vi "VelocityMeasure.vi"(5 "On/Off":bool, 6 "error in (no error)":errorcluster, 7 "Gray Image":T2, 8 "曝光时间/us":dbl, 9 "dpp/um":dbl) -> (0 "error out":errorcluster, 1 "粒子速度分布图":cluster{dbl[], i32[]}, 2 "实时速度":T1, 3 "平均速度":dbl format="%0.2f")   [LabVIEW 2012]
uses:
  <vilib>/vision/Image Controls.llb/IMAQ Image.ctl
  <vilib>/vision/NI_Vision_Development_Module.lvlib
  <vilib>/gmath/NI_Gmath.lvlib
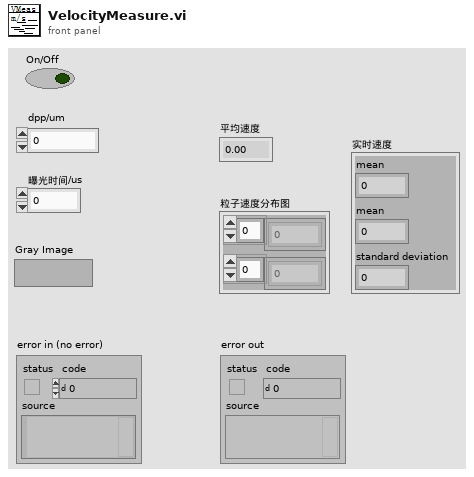
[diagram p1: front panel]
types:
  T1 = cluster{"mean":dbl, "mean":dbl, "standard deviation":dbl}
  T2 = typedef "IMAQ Image.ctl" = refnum<image>
  T3 = enum16{"arithmetic", "geometric", "harmonic", "trimmed", "median"}
  T4 = typedef "Particle Parameters" = i32
  T5 = cluster{"mean value":dbl, "mean value":dbl, "spread value":dbl}
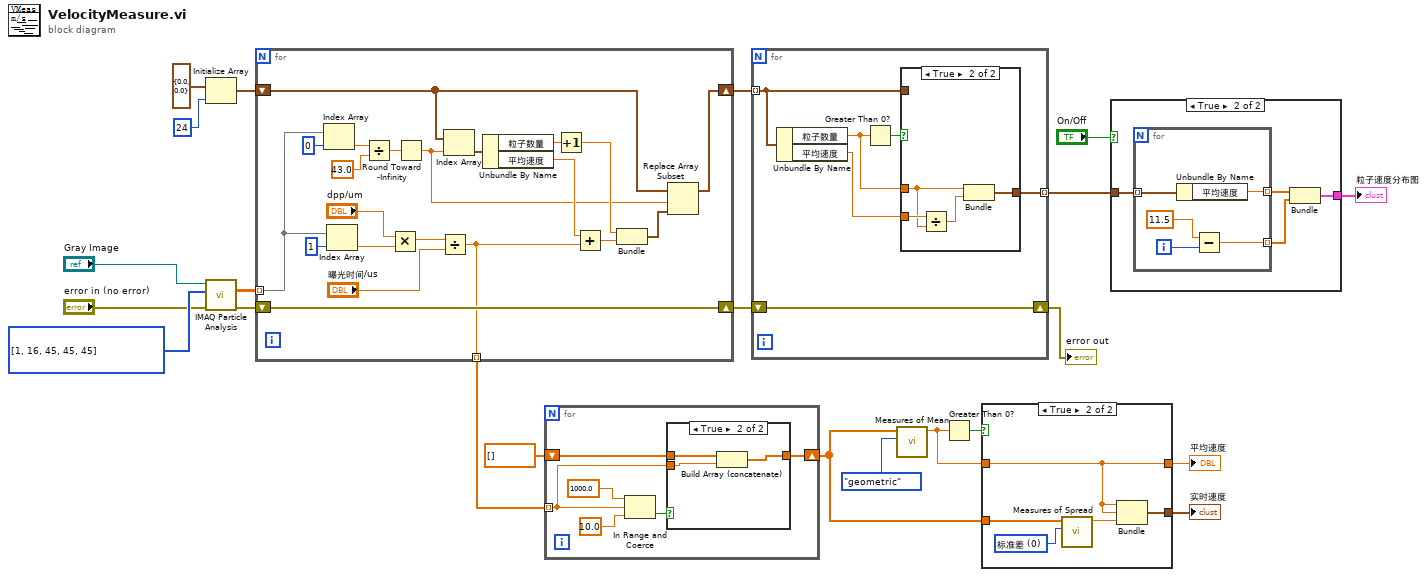
[diagram p0: block diagram]
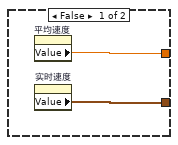
[diagram p2: hidden frame]
diagram:
  w22 = T4[] [1, 16, 45, 45, 45] items=["Center of Mass X", "Center of Mass Y", "First Pixel X", "First Pixel Y", "Bounding Rect Left", "Bounding Rect Top", "Bounding Rect Right", "Bounding Rect Bottom", "Max Feret Diameter Start X", "Max Feret Diameter Start Y", "Max Feret Diameter End X", "Max Feret Diameter End Y", "Max Horiz. Segment Length Left", "Max Horiz. Segment Length Right", "Max Horiz. Segment Length Row", "-", "Bounding Rect Width", "Bounding Rect Height", "Bounding Rect Diagonal", "Perimeter", "Convex Hull Perimeter", "Holes' Perimeter", "Max Feret Diameter", "Equivalent Ellipse Major Axis", "Equivalent Ellipse Minor Axis", "Equivalent Ellipse Minor Axis (Feret)", "Equivalent Rect Long Side", "Equivalent Rect Short Side", "Equivalent Rect Diagonal", "Equivalent Rect Short Side (Feret)", "Average Horiz. Segment Length", "Average Vert. Segment Length", "Hydraulic Radius", "Waddel Disk Diameter", "-", "Area", "Holes' Area", "Particle & Holes' Area", "Convex Hull Area", "Image Area", "-", "Number of Holes", "Number of Horiz. Segments", "Number of Vert. Segments", "-", "Orientation", "Max Feret Diameter Orientation", "-", "% Area/Image Area", "% Area/(Particle & Holes' Area)", "Ratio of Equivalent Ellipse Axes", "Ratio of Equivalent Rect Sides", "-", "Elongation Factor", "Compactness Factor", "Heywood Circularity Factor", "Type Factor", "-", "Sum X", "Sum Y", "Sum XX", "Sum XY", "Sum YY", "Sum XXX", "Sum XXY", "Sum XYY", "Sum YYY", "-", "Moment of Inertia XX", "Moment of Inertia XY", "Moment of Inertia YY", "Moment of Inertia XXX", "Moment of Inertia XXY", "Moment of Inertia XYY", "Moment of Inertia YYY", "Norm. Moment of Inertia XX", "Norm. Moment of Inertia XY", "Norm. Moment of Inertia YY", "Norm. Moment of Inertia XXX", "Norm. Moment of Inertia XXY", "Norm. Moment of Inertia XYY", "Norm. Moment of Inertia YYY", "Hu Moment 1", "Hu Moment 2", "Hu Moment 3", "Hu Moment 4", "Hu Moment 5", "Hu Moment 6", "Hu Moment 7"] ("Pixel Measurements")
  n1 = Initialize Array(cluster{"粒子数量":dbl, "平均速度":dbl} {"粒子数量"=0.0, "平均速度"=0.0} ("速度信号簇"), 24 ("维数大小")) -> (w19:cluster{"粒子数量":dbl, "平均速度":dbl}[])
  n2 = call "IMAQ Particle Analysis"("error in (no error)"="error in (no error)", "Pixel Measurements"=w22, "Image"="Gray Image") -> ("error out"=w17:errorcluster, "Particle Measurements (Pixels)"=w9:dbl[][])  [unwired: 3 in, 4 out]
  n3 = for {
    tunnel: w9 -> [w36] mode=indexing
    shift-right: [w27] -> w18
    shift-left: w19 -> [w28]
    shift-right: [w26] -> w16
    shift-left: w17 -> [w26]
    tunnel: [w23] -> w1 mode=indexing
    n4 = Index Array(array=w36, index=0 ("索引")) -> (element=w42:dbl)
    n5 = Index Array(array=w36, index=1 ("索引")) -> (element=w37:dbl)
    n6 = Divide(x=w42, y=43.0) -> (x/y=w40:dbl)
    n7 = Multiply(x="dpp/um", y=w37) -> (x*y=w25:dbl)
    n8 = Round Toward -Infinity(1:w40) -> (0:w29:dbl)
    n9 = Divide(x=w25, y="曝光时间/us") -> (x/y=w23:dbl)
    n10 = Index Array(array=w28, index=w29) -> (element=w35:cluster{"粒子数量":dbl, "平均速度":dbl})
    n11 = Unbundle By Name(w35) -> ("粒子数量"=w34:dbl, "平均速度"=w33:dbl)
    n12 = Increment(x=w34) -> (x+1=w32:dbl)
    n13 = Add(x=w33, y=w23) -> (x+y=w31:dbl)
    n14 = Bundle(w32, w31) -> (w30:cluster{dbl, dbl})  [unwired: 1 in]
    n15 = Replace Array Subset(array=w28, new element=w30, index=w29) -> (w27:cluster{"粒子数量":dbl, "平均速度":dbl}[])
  }
  n16 = for {
    shift-right: [w48] -> w3
    shift-left: dbl[] [] -> [w49]
    tunnel: w1 -> [w47] mode=indexing
    n17 = In Range and Coerce(upper limit=1000.0 ("上限"), x=w47, lower limit=10.0 ("下限")) -> (In Range?=w46:bool)  [unwired: 1 out]
    n18 = case shown="True" w46 {
      tunnel: w49 -> [w50 w53]
      tunnel: w47 -> [_ w52]
      tunnel: [w50 w51] -> w48
      frame False {
      }
      frame True {
        n19 = Build Array (concatenate)(w53, w52) -> (w51:dbl[])
      }
    }
  }
  n20 = for {
    tunnel: w18 -> [w57] mode=indexing
    tunnel: [w56] -> w14 mode=indexing
    shift-right: [w55] -> w15
    shift-left: w16 -> [w55]
    n21 = Unbundle By Name(w57) -> ("粒子数量"=w58:dbl, "平均速度"=w54:dbl)
    n22 = Greater Than 0?(x=w58) -> (x > 0?=w59:bool)
    n23 = case shown="True" w59 {
      tunnel: w54 -> [_ w64]
      tunnel: w58 -> [_ w63]
      tunnel: [w60 w62] -> w56
      tunnel: w57 -> [w60 _]
      frame False {
      }
      frame True {
        n24 = Divide(x=w64, y=w63) -> (x/y=w61:dbl)
        n25 = Bundle("粒子数量"=w63, w61) -> (w62:cluster{"粒子数量":dbl, dbl})  [unwired: 1 in]
      }
    }
  }
  "error out" <- w15
  n26 = call <vilib>:"Measures of Mean.vi"("type"=T3."geometric", "x array"=w3) -> ("mean value"=w2:dbl)  [unwired: 8 in, 1 out]
  n27 = Greater Than 0?(x=w2) -> (x > 0?=w8:bool)
  n28 = case shown="True" w8 {
    tunnel: w2 -> [_ w67]
    tunnel: w3 -> [_ w69]
    tunnel: [w66 w67] -> w7
    tunnel: [w65 w68] -> w6
    frame False {
      n29 = property on="平均速度" class="DigNum (strict)"() -> ("Value"=w66:dbl)  [unwired: 2 in, 2 out]
      n30 = property on="实时速度" class="Clust (strict)"() -> ("Value"=w65:T1)  [unwired: 2 in, 2 out]
    }
    frame True {
      w71 = 0 items=["标准差", "范围", "均值绝对偏差", "四分位数间距"] ("type")
      n31 = call <vilib>:"Measures of Spread.vi"("type"=w71, "x array"=w69) -> ("spread value"=w70:dbl)  [unwired: 8 in, 1 out]
      n32 = Bundle("mean value"=w67, "mean value"=w67, "spread value"=w70) -> (w68:T5)  [unwired: 1 in]
    }
  }
  "平均速度" <- w7
  "实时速度" <- w6
  n33 = case shown="True" "On/Off" {
    tunnel: w14 -> [_ w75]
    tunnel: [_ w73] -> w13
    frame False {
    }
    frame True {
      n34 = for {
        tunnel: w75 -> [w80] mode=indexing
        tunnel: [w79] -> w74 mode=indexing
        tunnel: [w77] -> w72 mode=indexing
        i -> [w76]
        n35 = Unbundle By Name(w80) -> ("平均速度"=w79:dbl)
        n36 = Subtract(x=11.5, y=w76) -> (x-y=w77:dbl)
      }
      n37 = Bundle(w74, w72) -> (w73:cluster{dbl[], dbl[]})  [unwired: 1 in]
    }
  }
  "粒子速度分布图" <- w13
